vi "Autonomous.vi"() -> (2 "Switch To Teleop":bool, 3 "output cluster":T1)   [LabVIEW 2014]
panel:
  in  "Was the goal lit?":string(combo)="No"
  in  "Did they move?":string(combo)="No"
  in  "SWITCH TO TELEOP":bool
  in  "Autonomous?":string(combo)="No"
  in  "Did they start in \nthe goalie zone??":string(combo)="No"
  in  "Autonomous Comments":string
  in  "Team Number":string
  in  "Bottom Goal":dbl
  in  "Top Goal":dbl
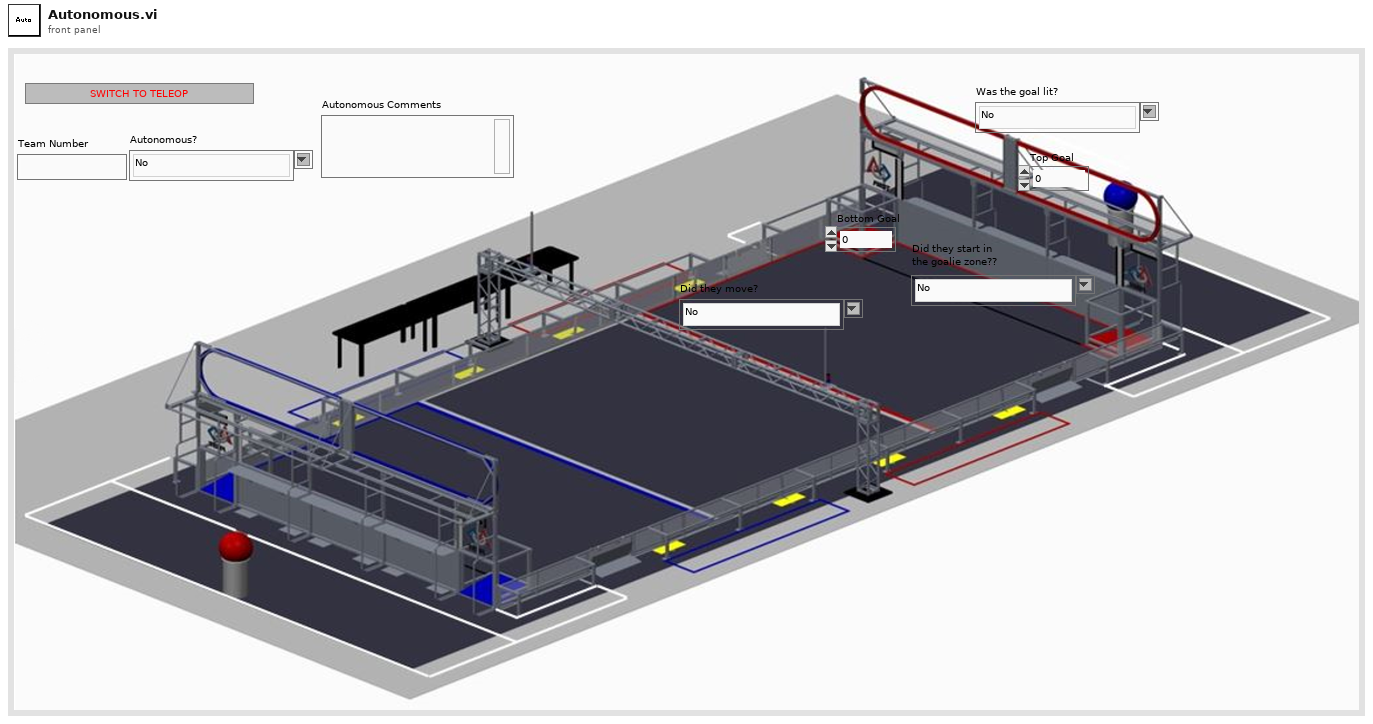
[diagram p1: front panel]
types:
  T1 = cluster{"Team Number":string, "Autonomous?":string, "Autonomous Comments":string, "Did they start in \nthe goalie zone??":string, "Top Goal":dbl, "Bottom Goal":dbl, "Did they move?":string, "Was the goal lit?":string}
  T2 = cluster{"Team Number":string, "Autonomous?":string, "Autonomous Comments":string, "Did they start in \nthe goalie zone??":string, dbl, dbl, "Did they move?":string, "Was the goal lit?":string}
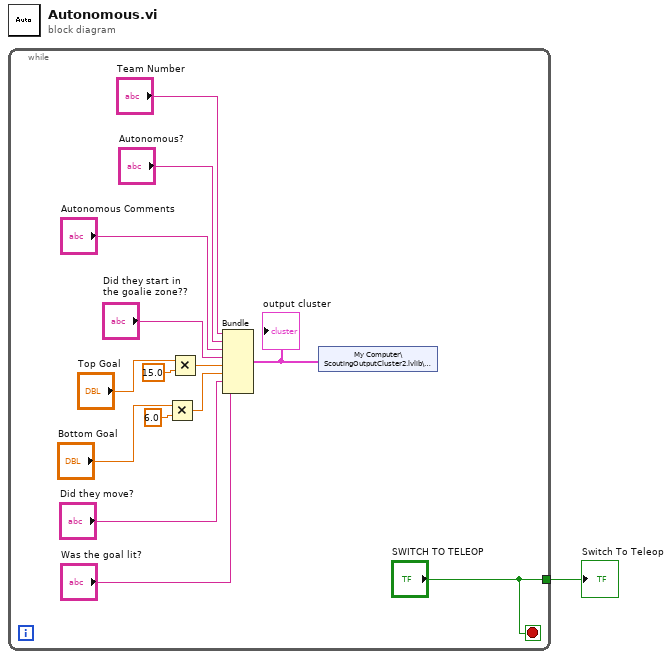
[diagram p0: block diagram]
diagram:
  n1 = while {
    tunnel: ["SWITCH TO TELEOP"] -> w1
    stop <- "SWITCH TO TELEOP" stop-if-true
    n2 = Multiply(x="Bottom Goal", y=6.0) -> (x*y=w6:dbl)
    n3 = Multiply(x="Top Goal", y=15.0) -> (x*y=w7:dbl)
    n4 = Bundle("Team Number"="Team Number", "Autonomous?"="Autonomous?", "Autonomous Comments"="Autonomous Comments", "Did they start in \nthe goalie zone??"="Did they start in \nthe goalie zone??", w7, w6, "Did they move?"="Did they move?", "Was the goal lit?"="Was the goal lit?") -> (w3:T2)  [unwired: 1 in]
    "output cluster" <- w3
    n5 = shared-variable "My Computer\\ScoutingOutputCluster2.lvlib\\output cluster"(w3) -> ()  [unwired: 1 in, 1 out]
  }
  "Switch To Teleop" <- w1
